vi "Tank.vi"   [LabVIEW 2012, in "Serenity_mk2.lvrbt"]
uses:
  Serenity_mk2.lvrbt
  <vilib>/NXT/Hardware/Plugins/Tetrix 180 deg Servo/Tetrix180ServoAddress.ctl
  <vilib>/NXT/Hardware/Plugins/Tetrix DC Motor/TetrixDCMotorAddress.ctl
  <vilib>/NXT/NXTIO Xnodes/NXTIONodeSubVIs/TETRIX IO Move Servos.vi
  <vilib>/NXT/NXTIO Xnodes/NXTIONodeSubVIs/TETRIX IO Move DC Motors.vi
  <vilib>/NXT/NXTIO Xnodes/NXTIONodeSubVIs/TETRIX IO Check Battery.vi
  <vilib>/NXT/NXTIO Xnodes/NXTIONodeSubVIs/TETRIX IO Stop DC Motors.vi
  <vilib>/NXT/Subs/LVHSConnector.ctl
  <vilib>/NXT/NXTIO Xnodes/AddressXNode/NXTIOAddress.xnode
  MecanumDrive/Mecanum Drive.lvrbt
  <vilib>/NXT/NXTIO Xnodes/NXTIOXNode/NXTIO.xnode
  <vilib>/NXT/LegoClasses/BrickReference/BrickReference.lvclass
panel:
  # "This VI was generated based on your configuration in the Remote Control Editor. You may modify the code as needed for your robot. To test this program for an FTC match, return to the Remote Control Editor, select the \"Run Program\" tab, and choose \"Teleop\"."
types:
  T1 = typedef "Tetrix180ServoAddress.ctl" = i32
  T2 = typedef "LVHSConnector.ctl" = refnum<class "BrickReference.lvclass">
  T3 = typedef "TetrixDCMotorAddress.ctl" = i32
  T4 = cluster{"TetrixDCMotor":T3, "TetrixDCMotor 2":T3}
  T5 = typedef "FTC ControllerState.ctl" = cluster{"Left X":i8, "Left Y":i8, "Right X":i8, "Right Y":i8, "Button Encoding 9-12":u8, "Button Encoding 1-8":u8, "POV":T6}
  T6 = typedef "FTC POVState.ctl" = i8
  T7 = typedef "FTC ButtonEventType.ctl" = enum16{"Pressed", "Released"}
  T8 = cluster{"Button ID":enum16{"None", "Button 1", "Button 2", "Button 3", "Button 4", "Button 5", "Button 6", "Button 7", "Button 8", "Button 9", "Button 10", "Button 11", "Button 12", "POV Up", "POV Up Right", "POV Right", "POV Down Right", "POV Down", "POV Down Left", "POV Left", "POV Up Left"}, "Event Type":T7}[]
  T9 = typedef "FTC ButtonState.ctl" = cluster{"Button 1":bool, "Button 2":bool, "Button 3":bool, "Button 4":bool, "Button 5":bool, "Button 6":bool, "Button 7":bool, "Button 8":bool, "Button 9":bool, "Button 10":bool, "Button 11":bool, "Button 12":bool, "POV":T6}
  T10 = enum16{"None", "Button 1", "Button 2", "Button 3", "Button 4", "Button 5", "Button 6", "Button 7", "Button 8", "Button 9", "Button 10", "Button 11", "Button 12", "POV Up", "POV Up Right", "POV Right", "POV Down Right", "POV Down", "POV Down Left", "POV Left", "POV Up Left"}
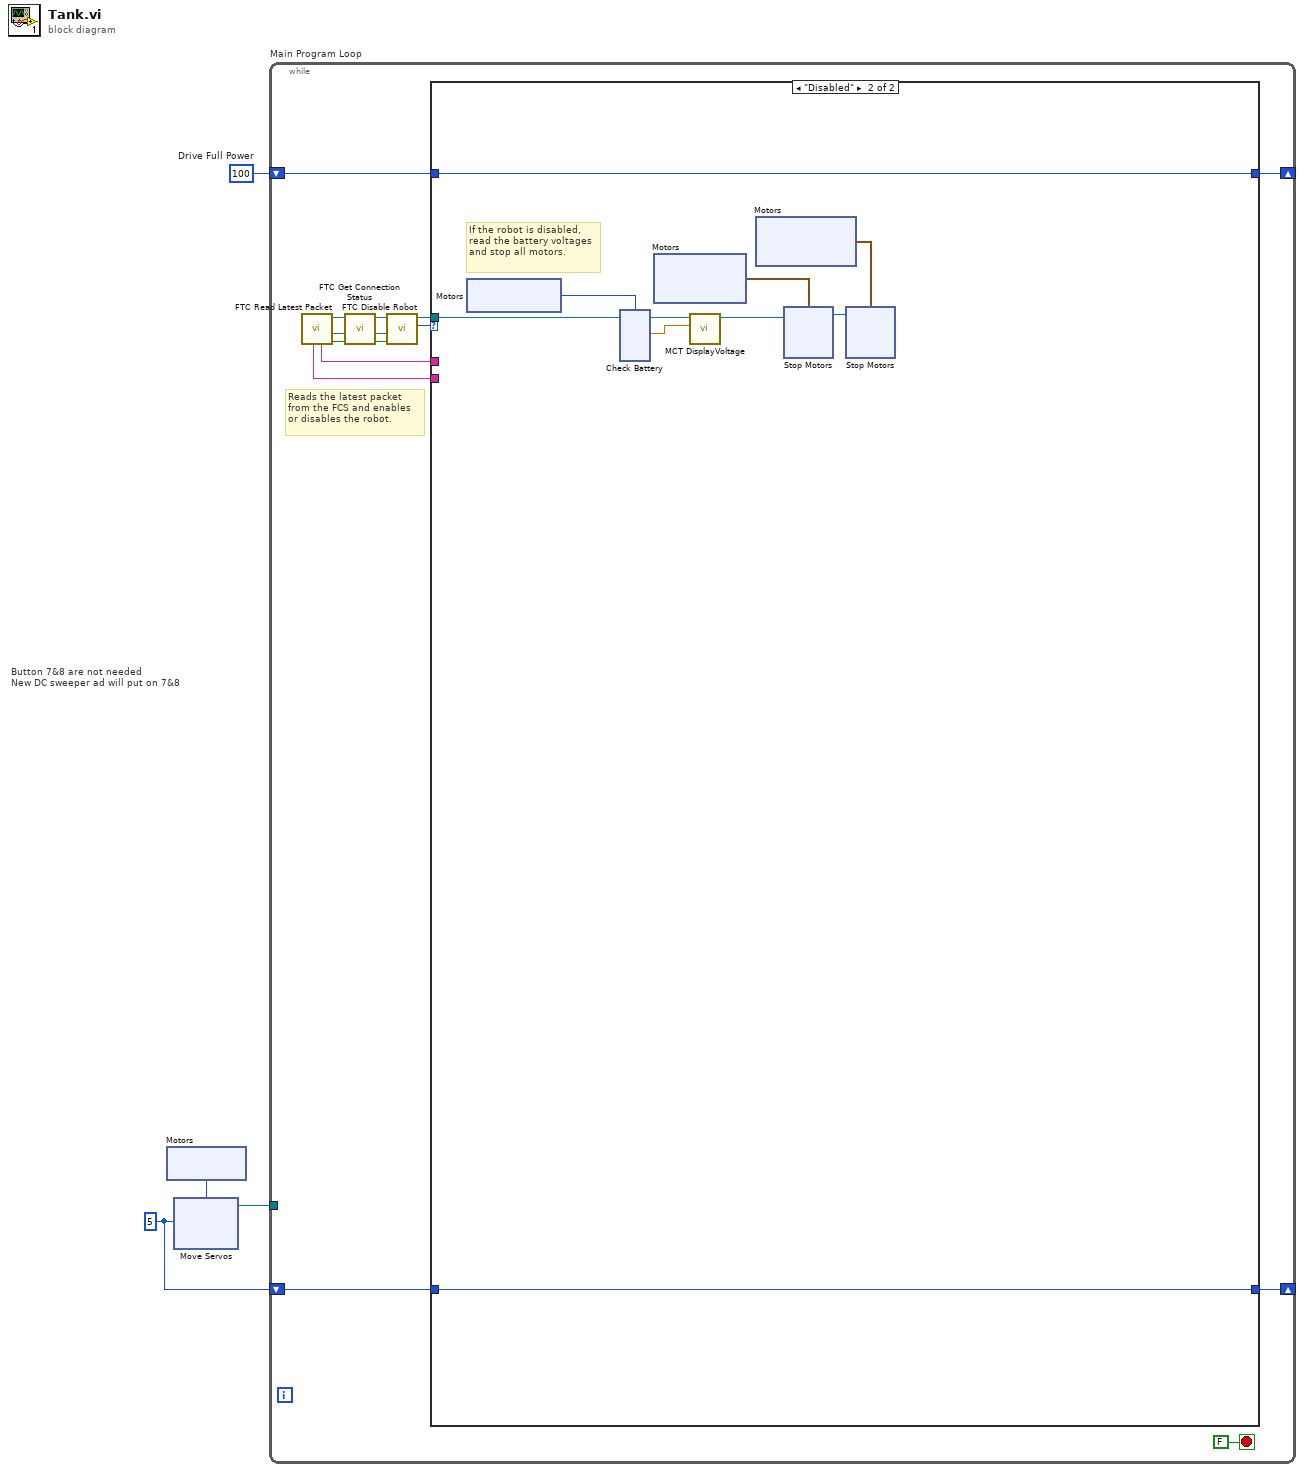
[diagram p0: block diagram]
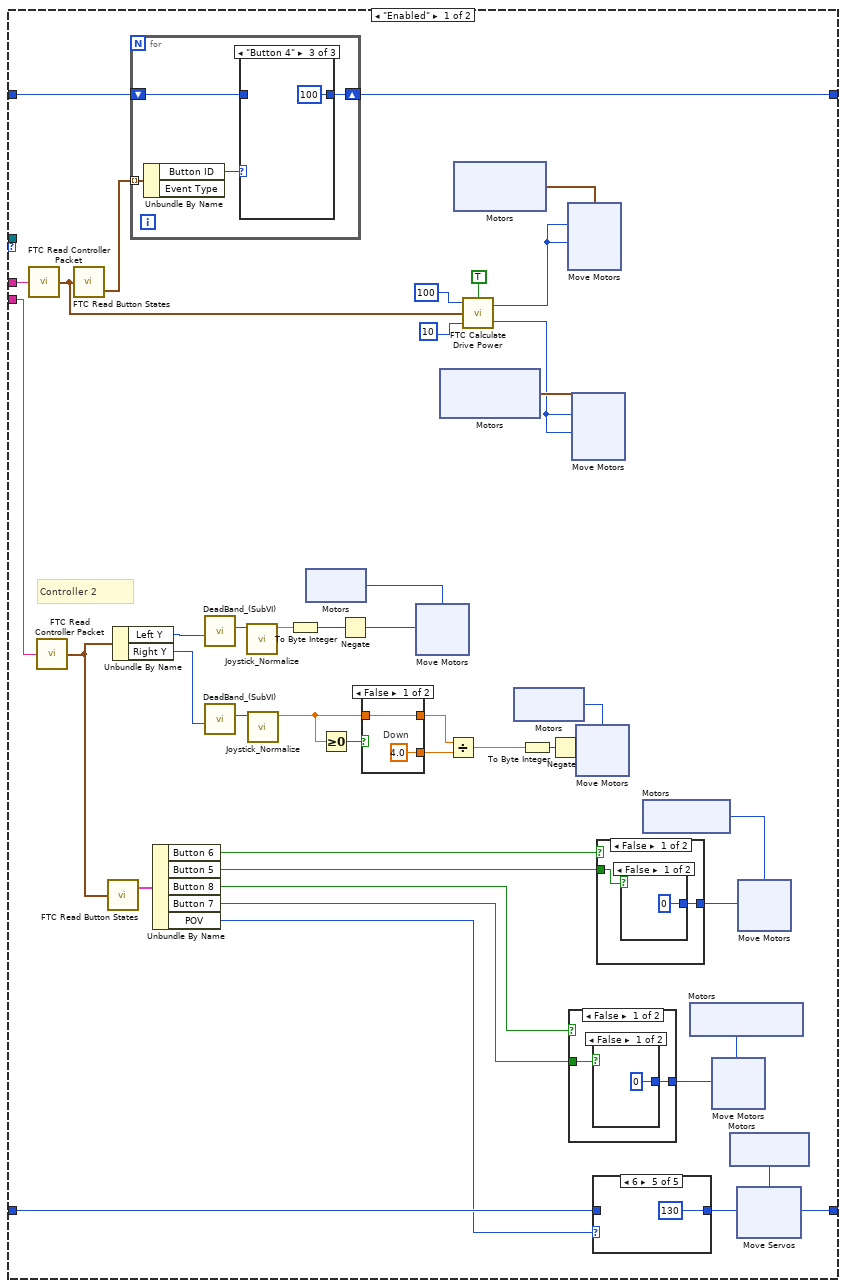
[diagram p2: hidden frame]
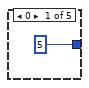
[diagram p3: hidden frame]
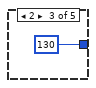
[diagram p5: hidden frame]
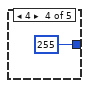
[diagram p6: hidden frame]
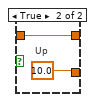
[diagram p7: hidden frame]
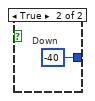
[diagram p8: hidden frame]
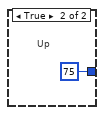
[diagram p9: hidden frame]
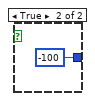
[diagram p10: hidden frame]
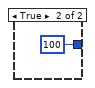
[diagram p11: hidden frame]
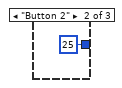
[diagram p13: hidden frame]
diagram:
  w1 = u8 5 ("Position 1")
  w4 = 100  # Drive Full Power
  # "Button 7&8 are not needed\nNew DC sweeper ad will put on 7&8"
  n1 = xnode "Motors"() -> ("Motor"=w2:T1)
  n2 = xnode "Move Servos"("Position 1"=w1, "Motors"=w2) -> ("NXT/EV3"=w3:T2)  [unwired: 1 in]
  n3 = while "Main Program Loop" {
    shift-right: [w7] -> _
    shift-left: w4 -> [w8]
    tunnel: w3 -> [_]
    shift-right: [w6] -> _
    shift-left: w1 -> [w5]
    stop <- FALSE stop-if-true
    # "Reads the latest packet\nfrom the FCS and enables\nor disables the robot."
    n4 = call <vilib>:"FTC Read Latest Packet.vi"() -> ("Packet Received?"=w16:bool, "Stopped?"=w13:bool, "NXT"=w15:T2, "Controller 1"=w18:string, "Controller 2"=w17:string)  [unwired: 6 in, 1 out]
    n5 = call <vilib>:"FTC Get Connection Status.vi"("Packet Received?"=w16, "Stopped?"=w13, "NXT"=w15) -> ("Online?"=w10:bool, "Stopped?"=w11:bool, "NXT"=w12:T2)  [unwired: 5 in]
    n6 = call <vilib>:"FTC Disable Robot.vi"("Online?"=w10, "Stopped?"=w11, "NXT"=w12) -> ("Enabled?"=w14:enum16{"Disabled", "Enabled"}, "NXT"=w9:T2)  [unwired: 3 in]
    n7 = case "disableCase" shown="\"Disabled\"" w14 {
      tunnel: w18 -> [w62 _]
      tunnel: w17 -> [w61 _]
      tunnel: w9 -> [_ w156]
      tunnel: w8 -> [w59 w148]
      tunnel: [w58 w148] -> w7
      tunnel: [w32 w147] -> w6
      tunnel: w5 -> [w35 w147]
      frame "Enabled" {
        # "Controller 2"
        n8 = call <vilib>:"FTC Read Controller Packet.vi"("Packet"=w62) -> ("Controller State"=w30:T5)  [unwired: 4 in]
        n9 = call <vilib>:"FTC Read Controller Packet.vi"("Packet"=w61) -> ("Controller State"=w56:T5)  [unwired: 4 in]
        n10 = call <vilib>:"FTC Read Button States.vi"("Controller State"=w30) -> ("Button Events"=w60:T8)  [unwired: 2 in, 1 out]
        n11 = call <vilib>:"FTC Read Button States.vi"("Controller State"=w56) -> ("Button States"=w34:T9)  [unwired: 2 in, 1 out]
        n12 = Unbundle By Name(w56) -> ("Left Y"=w20:i8, "Right Y"=w23:i8)
        n13 = for {
          tunnel: w60 -> [w143] mode=indexing
          shift-right: [w141] -> w58
          shift-left: w59 -> [w140]
          n14 = Unbundle By Name(w143) -> ("Button ID"=w142:T10)  [unwired: 1 out]
          n15 = case shown="\"Button 4\"" w142 {
            tunnel: [w144 25 100] -> w141
            tunnel: w140 -> [w144 _ _]
            frame "None", Default {
            }
            frame "Button 2" {
            }
            frame "Button 4" {
            }
          }
        }
        n16 = Unbundle By Name(w34) -> ("Button 6"=w53:bool, "Button 5"=w52:bool, "Button 8"=w48:bool, "Button 7"=w47:bool, "POV"=w33:T6)
        n17 = call "DeadBand_(SubVI).vi"("Axis In"=w20) -> ("Axis out"=w22:i8)  [unwired: 10 in]
        n18 = call "DeadBand_(SubVI).vi"("Axis In"=w23) -> ("Axis out"=w24:i8)  [unwired: 10 in]
        n19 = call "Joystick_Normalize.vi"("Joystick In"=w22) -> ("Norm Out"=w21:sgl)  [unwired: 10 in]
        n20 = call "Joystick_Normalize.vi"("Joystick In"=w24) -> ("Norm Out"=w42:sgl)  [unwired: 10 in]
        n21 = To Byte Integer(number=w21) -> (8bit integer=w44:i8)
        n22 = xnode "Motors"() -> ("Motor"=w57:T3)
        n23 = Greater Or Equal To 0?(x=w42) -> (x >= 0?=w38:bool)
        n24 = Negate(x=w44) -> (-x=w43:i8)
        n25 = case shown="False" w38 {
          tunnel: [w77 w79] -> w36
          tunnel: w42 -> [w77 w79]
          tunnel: [sgl 4.0 sgl 10.0] -> w37
          frame False {
            # "Down"
          }
          frame True {
            # "Up"
          }
        }
        n26 = xnode "Move Motors"("Power/Speed 1"=w43, "Motors"=w57) -> ()  [unwired: 1 in, 1 out]
        n27 = xnode ("Motors")() -> ("Motor"=w40:cluster{"TetrixDCMotor":T3, "TetrixDCMotor":T3})
        n28 = Divide(x=w36, y=w37) -> (x/y=w45:sgl)
        n29 = xnode ("Motors")() -> ("Motor"=w39:cluster{"TetrixDCMotor":T3, "TetrixDCMotor":T3})
        n30 = call-poly <vilib>:"FTC Calculate Drive Power.vi"("Reverse"=TRUE, "Deadband (10)"=i8 10, "Controller State"=w30, "Power Level (50)"=i8 100) -> ("Right Motor Power"=w26:i8, "Left Motor Power"=w27:i8)
        n31 = xnode "Motors"() -> ("Motor"=w55:T3)
        n32 = To Byte Integer(number=w45) -> (8bit integer=w54:i8)
        n33 = Negate(x=w54) -> (-x=w46:i8)
        n34 = xnode ("Move Motors")("Power/Speed 2"=w27, "Power/Speed 1"=w27, "Motors"=w39) -> ()  [unwired: 1 in, 1 out]
        n35 = case shown="False" w48 {
          tunnel: w47 -> [w106 _]
          tunnel: [w105 i8 75] -> w41
          frame False {
            n36 = case shown="False" w106 {
              tunnel: [i8 0 i8 -40] -> w105
              frame False {
              }
              frame True {
                # "Down"
              }
            }
          }
          frame True {
            # "Up"
          }
        }
        n37 = xnode ("Move Motors")("Power/Speed 2"=w26, "Power/Speed 1"=w26, "Motors"=w40) -> ()  [unwired: 1 in, 1 out]
        n38 = xnode "Move Motors"("Power/Speed 1"=w46, "Motors"=w55) -> ()  [unwired: 1 in, 1 out]
        n39 = case shown="6" w33 {
          tunnel: [u8 5 w72 u8 130 u8 255 u8 130] -> w32
          tunnel: w35 -> [_ w72 _ _ _]
          frame 0 {
          }
          frame 1, Default {
          }
          frame 2 {
          }
          frame 4 {
          }
          frame 6 {
          }
        }
        n40 = case shown="False" w53 {
          tunnel: w52 -> [w120 _]
          tunnel: [w119 i8 100] -> w50
          frame False {
            n41 = case shown="False" w120 {
              tunnel: [i8 0 i8 -100] -> w119
              frame False {
              }
              frame True {
              }
            }
          }
          frame True {
          }
        }
        n42 = xnode "Motors"() -> ("Motor"=w51:T3)
        n43 = xnode "Motors"() -> ("Motor"=w49:T3)
        n44 = xnode "Move Motors"("Power/Speed 1"=w41, "Motors"=w49) -> ()  [unwired: 1 in, 1 out]
        n45 = xnode "Motors"() -> ("Motor"=w31:T1)
        n46 = xnode "Move Servos"("Position 1"=w32, "Motors"=w31) -> ()  [unwired: 1 in, 1 out]
        n47 = xnode "Move Motors"("Power/Speed 1"=w50, "Motors"=w51) -> ()  [unwired: 1 in, 1 out]
      }
      frame "Disabled" {
        # "If the robot is disabled, read the battery voltages and stop all motors."
        n48 = xnode ("Motors")() -> ("Motor"=w155:T3)
        n49 = xnode ("Check Battery")("Motors"=w155, "NXT/EV3"=w156) -> ("Voltage 1"=w154:sgl, "NXT/EV3"=w153:T2)
        n50 = xnode "Motors"() -> ("Motor"=w152:cluster{"TetrixDCMotor":T3, "TetrixDCMotor":T3})
        n51 = call <vilib>:"MCT DisplayVoltage.vi"("Motor Voltage"=w154, "NXT"=w153) -> ("NXT"=w151:T2)  [unwired: 9 in]
        n52 = xnode "Motors"() -> ("Motor"=w150:cluster{"TetrixDCMotor":T3, "TetrixDCMotor":T3})
        n53 = xnode "Stop Motors"("Motors"=w152, "NXT/EV3"=w151) -> ("NXT/EV3"=w149:T2)
        n54 = xnode "Stop Motors"("Motors"=w150, "NXT/EV3"=w149) -> ()  [unwired: 1 out]
      }
    }
  }
